vi "UTILITY Initialize Front Panel Controls.vi"(11 "Initial DOE Config":path=path "C:/GE/Washer DOE 6") -> (3 "Initial DOE Config 2":path, 6 "Front Panel Controls DOE":T1)   [LabVIEW 2019]
uses:
  Washer DOE/Type Definitions/DOE Front Panel Controls.ctl
  <vilib>/Utility/error.llb/whitespace.ctl
  <vilib>/Utility/file.llb/Read Delimited Spreadsheet (string).vi
panel:
  out "file or folder exists?":bool
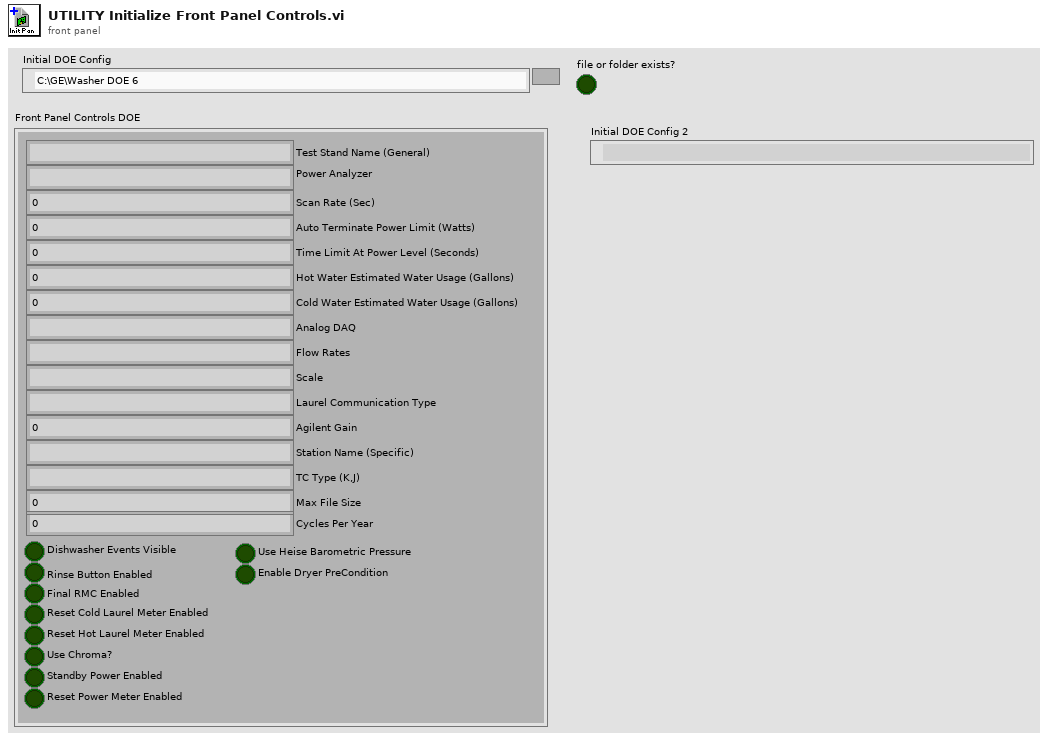
[diagram p1: front panel]
types:
  T1 = typedef "DOE Front Panel Controls.ctl" = cluster{"Test Stand Name (General)":string, "Power Analyzer":string, "Scan Rate (Sec)":dbl, "Auto Terminate Power Limit (Watts)":dbl, "Time Limit At Power Level (Seconds)":dbl, "Hot Water Estimated Water Usage (Gallons)":dbl, "Cold Water Estimated Water Usage (Gallons)":dbl, "Analog DAQ":string, "Flow Rates":string, "Scale":string, "Dishwasher Events Visible":bool, "Rinse Button Enabled":bool, "Final RMC Enabled":bool, "Reset Cold Laurel Meter Enabled":bool, "Laurel Communication Type":string, "Agilent Gain":dbl, "Station Name (Specific)":string, "TC Type (K,J)":string, "Max File Size":dbl, "Reset Hot Laurel Meter Enabled":bool, "Use Chroma?":bool, "Standby Power Enabled":bool, "Reset Power Meter Enabled":bool, "Use Heise Barometric Pressure":bool, "Enable Dryer PreCondition":bool, "Cycles Per Year":u32}
  T2 = typedef "whitespace.ctl" = u16
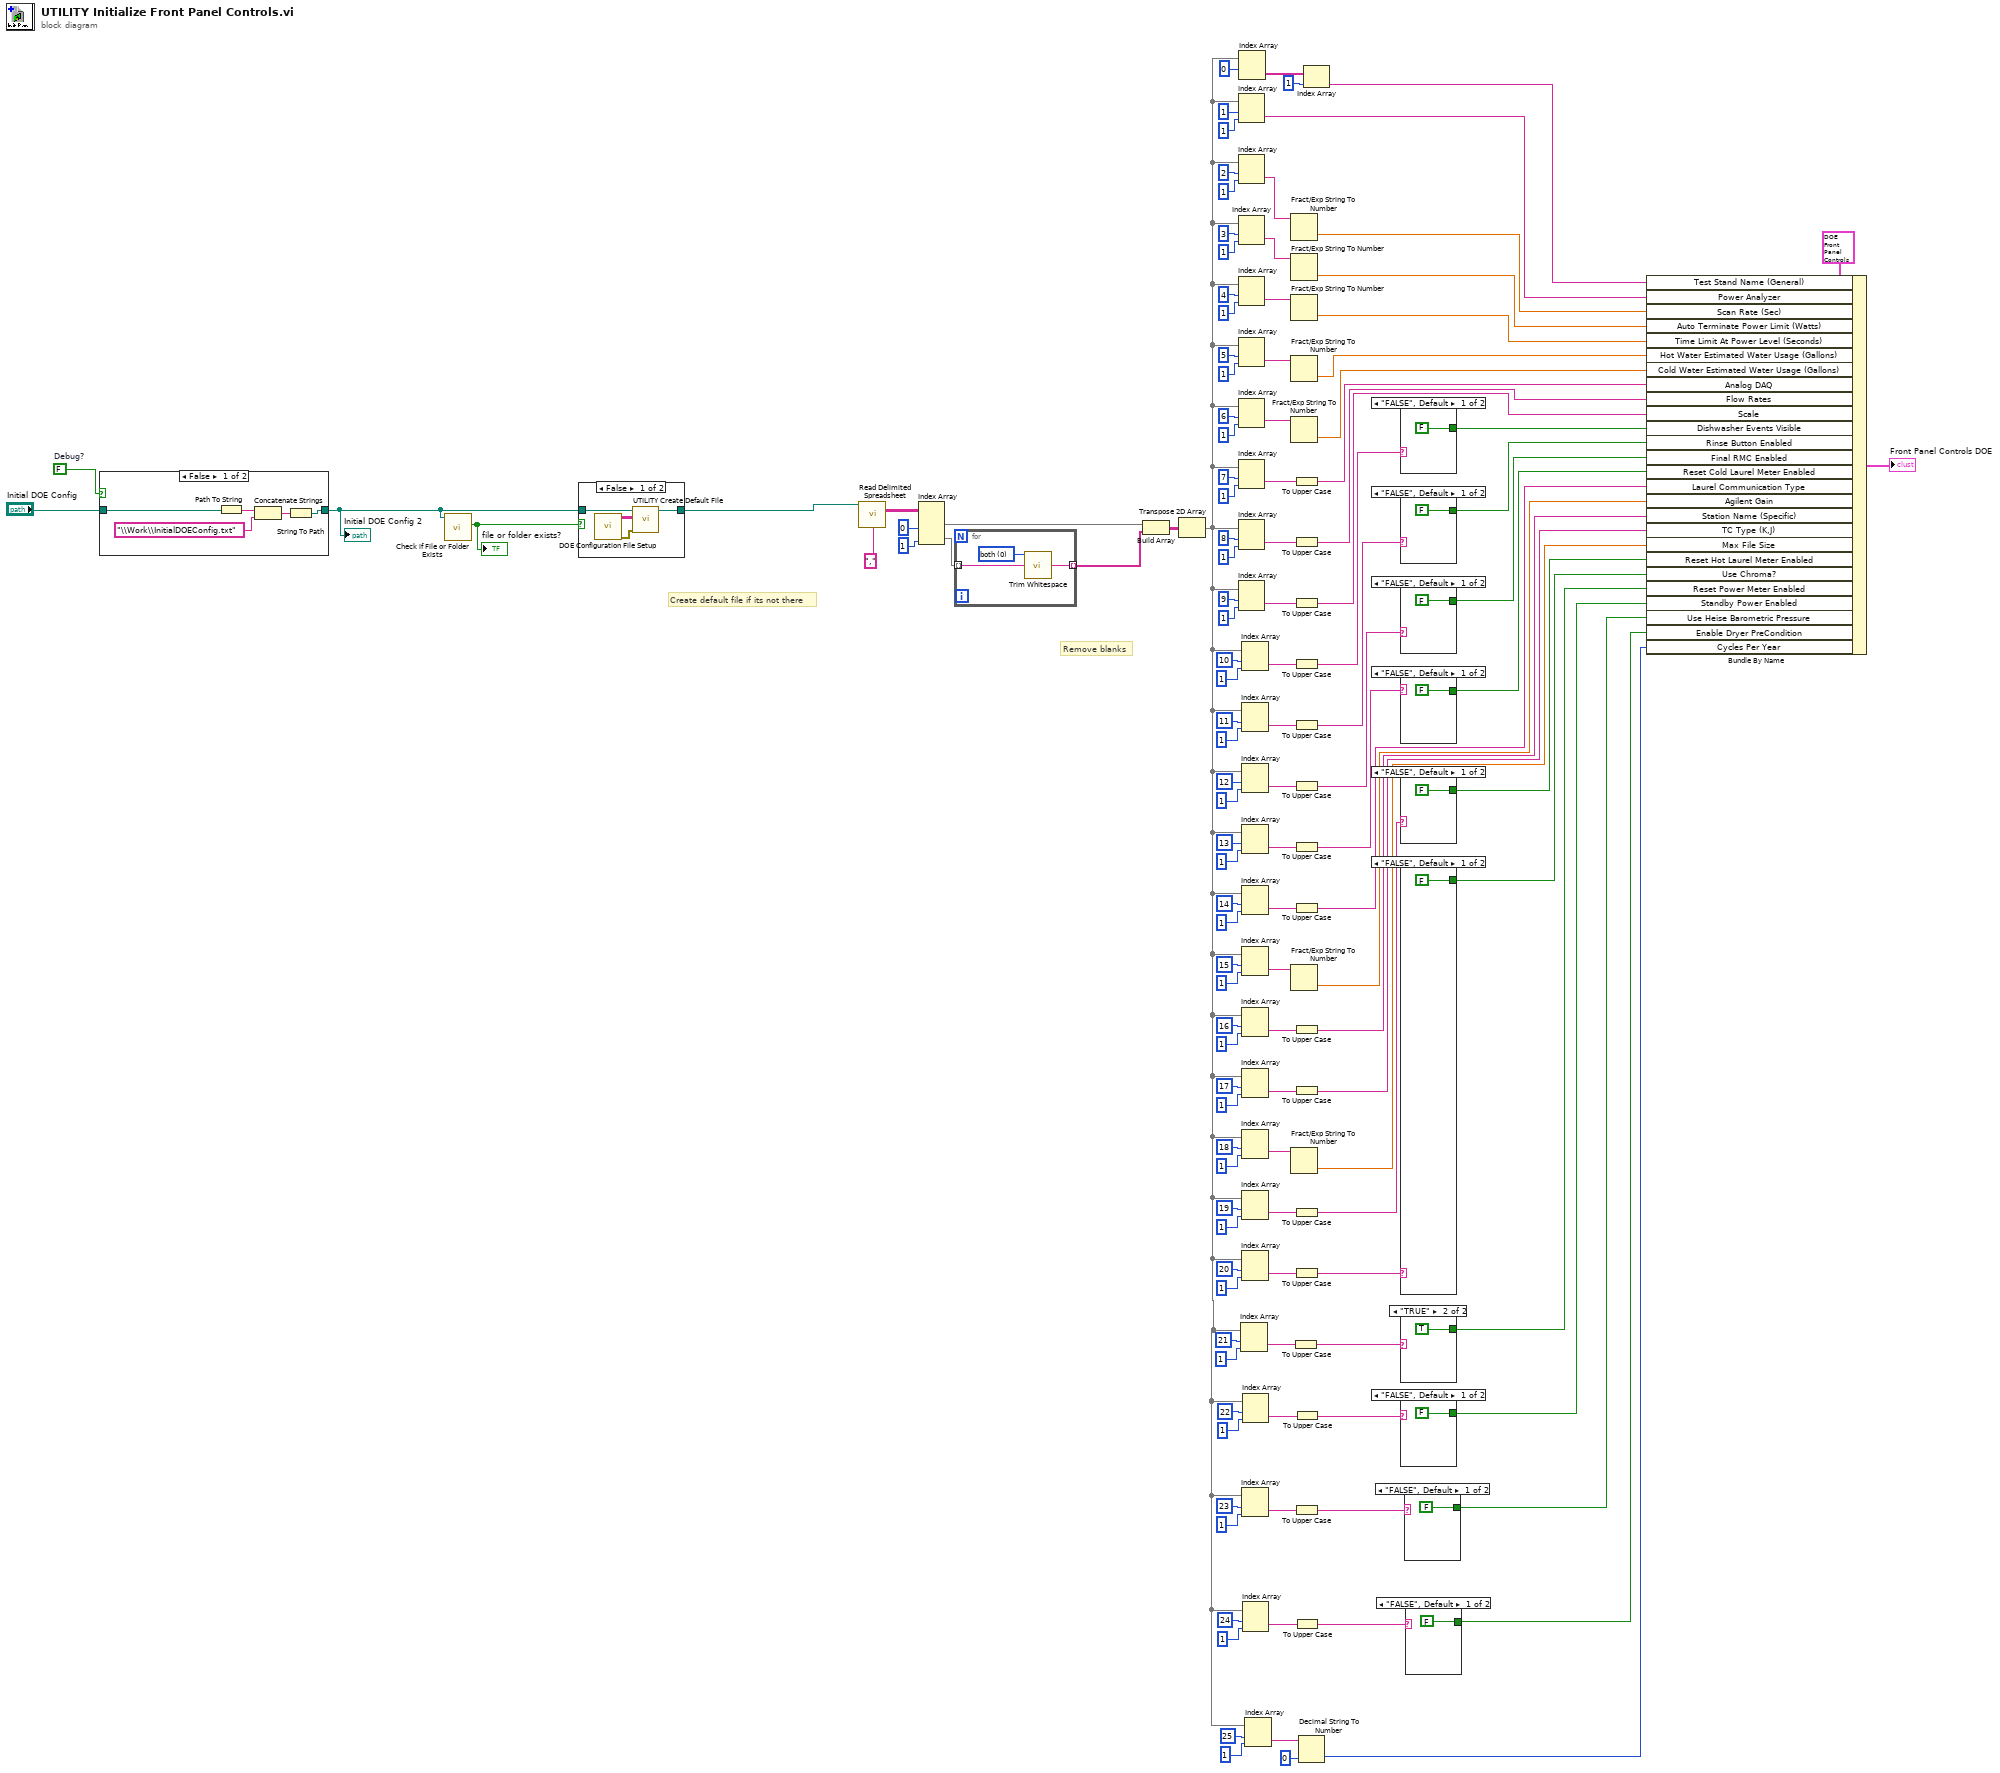
[diagram p0: block diagram]
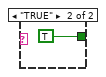
[diagram p2: hidden frame]
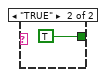
[diagram p3: hidden frame]
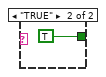
[diagram p4: hidden frame]
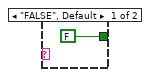
[diagram p5: hidden frame]
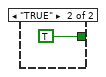
[diagram p6: hidden frame]
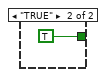
[diagram p7: hidden frame]
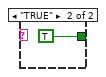
[diagram p9: hidden frame]
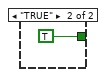
[diagram p10: hidden frame]
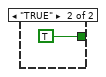
[diagram p11: hidden frame]
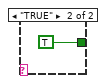
[diagram p12: hidden frame]
diagram:
  w52 = FALSE  # Debug?
  # "Remove blanks"
  # "Create default file if its not there"
  n1 = case shown="False" w52 {
    tunnel: "Initial DOE Config" -> [w135 w136]
    tunnel: [w131 w136] -> w45
    frame False {
      n2 = Path To String(path=w135) -> (string=w134:string)
      n3 = Concatenate Strings(w134, "\\Work\\InitialDOEConfig.txt") -> (w132:string)
      n4 = String To Path(string=w132) -> (path=w131:path)
    }
    frame True {
    }
  }
  "Initial DOE Config 2" <- w45
  n5 = call <vilib>:"Check if File or Folder Exists.vi"("path"=w45) -> ("file or folder exists?"=w109:bool)  [unwired: 8 in, 2 out]
  "file or folder exists?" <- w109
  n6 = case shown="False" w109 {
    tunnel: w45 -> [w140 w141]
    tunnel: [w139 w141] -> w3
    frame False {
      n7 = call "DOE Configuration File Setup.vi"() -> ("Error Out"=w138:errorcluster, "Config File"=w137:string[][])  [unwired: 10 in]
      n8 = call "UTILITY Create Default File.vi"("Error In"=w138, "Default File"=w137, "Initial DOE Config"=w140) -> ("new file path (Not A Path if cancelled)"=w139:path)  [unwired: 7 in, 1 out]
    }
    frame True {
    }
  }
  n9 = call-poly <vilib>:"Read Delimited Spreadsheet.vi"("file path (dialog if empty)"=w3, "delimiter (\\t)"="," ("delimiter (\\t)")) -> ("all rows"=w2:string[][])  [unwired: 8 in, 5 out]
  n10 = Index Array(array=w2, index (col) #1=0 ("disabled index (col)"), index (col) #2=1 ("disabled index (col)")) -> (element #1=w47:string[], element #2=w49:string[])  [unwired: 2 in]
  n11 = for {
    tunnel: w49 -> [w144] mode=indexing
    tunnel: [w142] -> w48 mode=indexing
    w143 = T2 0 items=["both", "start of string", "end of string"] ("location (both)")
    n12 = call <vilib>:"Trim Whitespace.vi"("string"=w144, "location (both)"=w143) -> ("trimmed string"=w142:string)
  }
  n13 = Build Array(w47, w48) -> (w46:string[][])
  n14 = Transpose 2D Array(2D array=w46) -> (transposed array=w8:string[][])
  n15 = Index Array(array=w8, index (row)=1 ("disabled index (row)"), index (col)=1 ("disabled index (col)")) -> (element=w123:string)
  n16 = Index Array(array=w8, index (row)=2 ("disabled index (row)"), index (col)=1 ("disabled index (col)")) -> (element=w118:string)
  n17 = Index Array(array=w8, index (row)=3 ("disabled index (row)"), index (col)=1 ("disabled index (col)")) -> (element=w117:string)
  n18 = Index Array(array=w8, index (row)=4 ("disabled index (row)"), index (col)=1 ("disabled index (col)")) -> (element=w116:string)
  n19 = Index Array(array=w8, index (row)=5 ("disabled index (row)"), index (col)=1 ("disabled index (col)")) -> (element=w103:string)
  n20 = Index Array(array=w8, index (row)=6 ("disabled index (row)"), index (col)=1 ("disabled index (col)")) -> (element=w104:string)
  n21 = Index Array(array=w8, index (row)=7 ("disabled index (row)"), index (col)=1 ("disabled index (col)")) -> (element=w70:string)
  n22 = Index Array(array=w8, index (row)=8 ("disabled index (row)"), index (col)=1 ("disabled index (col)")) -> (element=w69:string)
  n23 = Index Array(array=w8, index (row)=9 ("disabled index (row)"), index (col)=1 ("disabled index (col)")) -> (element=w67:string)
  n24 = Index Array(array=w8, index (row)=0) -> (element=w127:string[])  [unwired: 1 in]
  n25 = Index Array(array=w8, index (row)=21 ("disabled index (row)"), index (col)=1 ("disabled index (col)")) -> (element=w30:string)
  n26 = Index Array(array=w8, index (row)=10 ("disabled index (row)"), index (col)=1 ("disabled index (col)")) -> (element=w85:string)
  n27 = Index Array(array=w8, index (row)=11 ("disabled index (row)"), index (col)=1 ("disabled index (col)")) -> (element=w80:string)
  n28 = Index Array(array=w8, index (row)=12 ("disabled index (row)"), index (col)=1 ("disabled index (col)")) -> (element=w79:string)
  n29 = Index Array(array=w8, index (row)=13 ("disabled index (row)"), index (col)=1 ("disabled index (col)")) -> (element=w78:string)
  n30 = Index Array(array=w8, index (row)=14 ("disabled index (row)"), index (col)=1 ("disabled index (col)")) -> (element=w74:string)
  n31 = Index Array(array=w8, index (row)=15 ("disabled index (row)"), index (col)=1 ("disabled index (col)")) -> (element=w65:string)
  n32 = Index Array(array=w8, index (row)=16 ("disabled index (row)"), index (col)=1 ("disabled index (col)")) -> (element=w58:string)
  n33 = Index Array(array=w8, index (row)=17 ("disabled index (row)"), index (col)=1 ("disabled index (col)")) -> (element=w56:string)
  n34 = Index Array(array=w8, index (row)=18 ("disabled index (row)"), index (col)=1 ("disabled index (col)")) -> (element=w42:string)
  n35 = Index Array(array=w8, index (row)=19 ("disabled index (row)"), index (col)=1 ("disabled index (col)")) -> (element=w40:string)
  n36 = Index Array(array=w8, index (row)=20 ("disabled index (row)"), index (col)=1 ("disabled index (col)")) -> (element=w33:string)
  n37 = Index Array(array=w8, index (row)=23 ("disabled index (row)"), index (col)=1 ("disabled index (col)")) -> (element=w19:string)
  n38 = Index Array(array=w8, index (row)=22 ("disabled index (row)"), index (col)=1 ("disabled index (col)")) -> (element=w25:string)
  n39 = Index Array(array=w8, index (row)=24 ("disabled index (row)"), index (col)=1 ("disabled index (col)")) -> (element=w13:string)
  n40 = Index Array(array=w8, index (row)=25 ("disabled index (row)"), index (col)=1 ("disabled index (col)")) -> (element=w7:string)
  n41 = Fract/Exp String To Number(string=w118) -> (number=w113:dbl)  [unwired: 3 in, 1 out]
  n42 = Fract/Exp String To Number(string=w117) -> (number=w112:dbl)  [unwired: 3 in, 1 out]
  n43 = Fract/Exp String To Number(string=w116) -> (number=w111:dbl)  [unwired: 3 in, 1 out]
  n44 = Fract/Exp String To Number(string=w103) -> (number=w102:dbl)  [unwired: 3 in, 1 out]
  n45 = Fract/Exp String To Number(string=w104) -> (number=w101:dbl)  [unwired: 3 in, 1 out]
  n46 = Fract/Exp String To Number(string=w65) -> (number=w62:dbl)  [unwired: 3 in, 1 out]
  n47 = Fract/Exp String To Number(string=w42) -> (number=w41:dbl)  [unwired: 3 in, 1 out]
  n48 = To Upper Case(1:w30) -> (0:w24:string)
  n49 = To Upper Case(1:w70) -> (0:w4:string)
  n50 = To Upper Case(1:w69) -> (0:w68:string)
  n51 = To Upper Case(1:w67) -> (0:w66:string)
  n52 = To Upper Case(1:w85) -> (0:w84:string)
  n53 = To Upper Case(1:w80) -> (0:w83:string)
  n54 = To Upper Case(1:w79) -> (0:w82:string)
  n55 = To Upper Case(1:w78) -> (0:w81:string)
  n56 = To Upper Case(1:w74) -> (0:w71:string)
  n57 = To Upper Case(1:w58) -> (0:w57:string)
  n58 = To Upper Case(1:w56) -> (0:w53:string)
  n59 = To Upper Case(1:w40) -> (0:w37:string)
  n60 = To Upper Case(1:w33) -> (0:w32:string)
  n61 = To Upper Case(1:w19) -> (0:w20:string)
  n62 = To Upper Case(1:w25) -> (0:w23:string)
  n63 = To Upper Case(1:w13) -> (0:w12:string)
  n64 = Decimal String To Number(string=w7, default (0L)=u32 0 ("default (0 I32)")) -> (number=w6:u32)  [unwired: 1 in, 1 out]
  n65 = Index Array(array=w127, index=1) -> (element=w110:string)
  n66 = case shown="\"FALSE\", Default" w84 {
    tunnel: [FALSE TRUE] -> w86
    frame "FALSE", Default {
    }
    frame "TRUE" {
    }
  }
  n67 = case shown="\"FALSE\", Default" w83 {
    tunnel: [FALSE TRUE] -> w77
    frame "FALSE", Default {
    }
    frame "TRUE" {
    }
  }
  n68 = case shown="\"FALSE\", Default" w82 {
    tunnel: [FALSE TRUE] -> w76
    frame "FALSE", Default {
    }
    frame "TRUE" {
    }
  }
  n69 = case shown="\"FALSE\", Default" w81 {
    tunnel: [FALSE TRUE] -> w75
    frame "FALSE", Default {
    }
    frame "TRUE" {
    }
  }
  n70 = case shown="\"FALSE\", Default" w37 {
    tunnel: [FALSE TRUE] -> w36
    frame "FALSE", Default {
    }
    frame "TRUE" {
    }
  }
  n71 = case shown="\"FALSE\", Default" w32 {
    tunnel: [FALSE TRUE] -> w31
    frame "FALSE", Default {
    }
    frame "TRUE" {
    }
  }
  n72 = case shown="\"TRUE\"" w24 {
    tunnel: [FALSE TRUE] -> w22
    frame "FALSE", Default {
    }
    frame "TRUE" {
    }
  }
  n73 = case shown="\"FALSE\", Default" w23 {
    tunnel: [FALSE TRUE] -> w21
    frame "FALSE", Default {
    }
    frame "TRUE" {
    }
  }
  n74 = case shown="\"FALSE\", Default" w20 {
    tunnel: [FALSE TRUE] -> w16
    frame "FALSE", Default {
    }
    frame "TRUE" {
    }
  }
  n75 = case shown="\"FALSE\", Default" w12 {
    tunnel: [FALSE TRUE] -> w11
    frame "FALSE", Default {
    }
    frame "TRUE" {
    }
  }
  n76 = Bundle By Name(cluster=T1 {"Test Stand Name (General)"="", "Power Analyzer"="", "Scan Rate (Sec)"=0.0, "Auto Terminate Power Limit (Watts)"=0.0, "Time Limit At Power Level (Seconds)"=0.0, "Hot Water Estimated Water Usage (Gallons)"=0.0, "Cold Water Estimated Water Usage (Gallons)"=0.0, "Analog DAQ"="", "Flow Rates"="", "Scale"="", "Dishwasher Events Visible"=FALSE, "Rinse Button Enabled"=FALSE, "Final RMC Enabled"=FALSE, "Reset Cold Laurel Meter Enabled"=FALSE, "Laurel Communication Type"="", "Agilent Gain"=0.0, "Station Name (Specific)"="", "TC Type (K,J)"="", "Max File Size"=0.0, "Reset Hot Laurel Meter Enabled"=FALSE, "Use Chroma?"=FALSE, "Standby Power Enabled"=FALSE, "Reset Power Meter Enabled"=FALSE, "Use Heise Barometric Pressure"=FALSE, "Enable Dryer PreCondition"=FALSE, "Cycles Per Year"=0} ("Front Panel Controls DOE 2"), "Test Stand Name (General)"=w110, "Power Analyzer"=w123, "Scan Rate (Sec)"=w113, "Auto Terminate Power Limit (Watts)"=w112, "Time Limit At Power Level (Seconds)"=w111, "Hot Water Estimated Water Usage (Gallons)"=w102, "Cold Water Estimated Water Usage (Gallons)"=w101, "Analog DAQ"=w4, "Flow Rates"=w68, "Scale"=w66, "Dishwasher Events Visible"=w86, "Rinse Button Enabled"=w77, "Final RMC Enabled"=w76, "Reset Cold Laurel Meter Enabled"=w75, "Laurel Communication Type"=w71, "Agilent Gain"=w62, "Station Name (Specific)"=w57, "TC Type (K,J)"=w53, "Max File Size"=w41, "Reset Hot Laurel Meter Enabled"=w36, "Use Chroma?"=w31, "Reset Power Meter Enabled"=w22, "Standby Power Enabled"=w21, "Use Heise Barometric Pressure"=w16, "Enable Dryer PreCondition"=w11, "Cycles Per Year"=w6) -> (→"Front Panel Controls DOE":T1)
